vi "Update Tile.vi"(5 "Turn Direction":T1, 6 "Current Location":T3, 7 "Next Location":T3, 8 "Next State for Current Item":T2=1 items=["Empty", "Portal", "Open", "Wall", ">", "<", ">-^", ">-v", "^-<", "v-<"], 9 "Board Map in":T2[][](array[typedef]) items=["Empty", "Portal", "Open", "Wall", ">", "<", ">-^", ">-v", "^-<", "v-<"]) -> (3 "Board Map out":T2[][](array[typedef]) items=["Empty", "Portal", "Open", "Wall", ">", "<", ">-^", ">-v", "^-<", "v-<"], 4 "Next Direction":T1)   [LabVIEW 2020, in "AoC 2022.lvlib"]
uses:
  AoC 2022.lvlib
  Map Tile.ctl
  Day 15 - Beacon Exclusion Zone/private/Location.ctl
  Map Direction.ctl
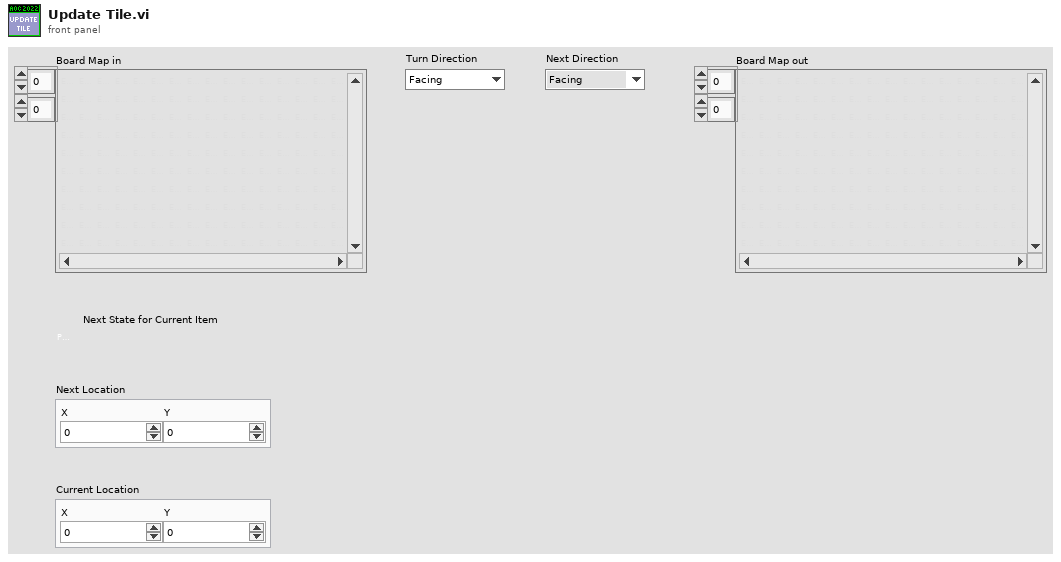
[diagram p1: front panel]
types:
  T1 = typedef "AoC 2022.lvlib/Map Direction.ctl" = enum16{"Facing", "Right", "Left", "Up", "Down"}
  T2 = typedef "AoC 2022.lvlib/Map Tile.ctl" = u16
  T3 = typedef "AoC 2022.lvlib/Location.ctl" = cluster{"X":i32, "Y":i32}
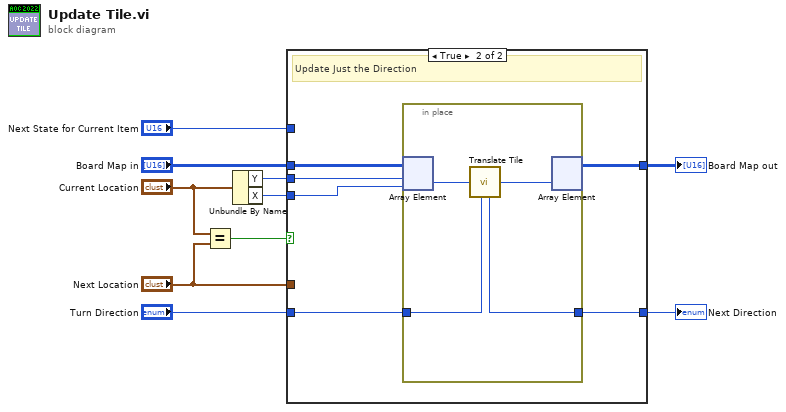
[diagram p0: block diagram]
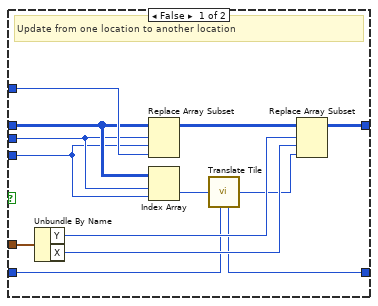
[diagram p2: hidden frame]
diagram:
  n1 = Equal?(x="Current Location", y="Next Location") -> (x = y?=w7:bool)
  n2 = Unbundle By Name("Current Location") -> ("Y"=w4:i32, "X"=w3:i32)
  n3 = case shown="True" w7 {
    tunnel: [w23 w29] -> w10
    tunnel: "Board Map in" -> [w17 w28]
    tunnel: "Next Location" -> [w22 _]
    tunnel: "Turn Direction" -> [w12 w27]
    tunnel: w4 -> [w16 w26]
    tunnel: w3 -> [w15 w25]
    tunnel: "Next State for Current Item" -> [w18 _]
    tunnel: [w11 w24] -> w1
    frame False {
      # "Update from one location to another location"
      n4 = Unbundle By Name(w22) -> ("Y"=w21:i32, "X"=w20:i32)
      n5 = Replace Array Subset(array=w17, new element=w18, index (row)=w16, index (col)=w15) -> (w19:T2[][])
      n6 = Index Array(array=w17, index (row)=w16, index (col)=w15) -> (element=w14:T2)
      n7 = call "Translate Tile.vi"("Tile in"=w14, "Direction in"=w12) -> ("Direction out"=w11:T1, "Tile out"=w13:T2)
      n8 = Replace Array Subset(array=w19, new element=w13, index (row)=w21, index (col)=w20) -> (w23:T2[][])
    }
    frame True {
      # "Update Just the Direction"
      n9 = in-place {
        in-place-border: w27 -> [w33]
        in-place-border: [w30] -> w24
        n10 = in-place-array #1(w28, w26, w25) -> (w31:T2)
        n11 = call "Translate Tile.vi"("Tile in"=w31, "Direction in"=w33) -> ("Direction out"=w30:T1, "Tile out"=w32:T2)
        n12 = in-place-array #1(w32) -> (w29:T2[][])  [unwired: 2 out]
      }
    }
  }
  "Board Map out" <- w10
  "Next Direction" <- w1
